vi "KM_FrequencyScan.vi"() -> ()   [LabVIEW 2015]
uses:
  MQM Data Transfer_KM.vi
  <vilib>/Utility/file.llb/Write To Spreadsheet File (string).vi
  <vilib>/Utility/file.llb/Write To Spreadsheet File (DBL).vi
  String Array Select.vi
  Numeric Array Select.vi
  plot refs -- filter related.ctl
  wavepacket.ctl
  filter method control.ctl
  peak -- parameters -- complex fit.ctl
  circle corners.ctl
  lorentzian.ctl
panel:
  out "cp lorentzian":T1={"Amplitude"=-1.0311345636926572, "omega(0)"=-1.0311345636926572, "Gamma"=-1.0311345636926572, "phase"=-1.0311345636926572, "Q"=-1.0311345636926572, "Norm  Ampl"=-1.0311345636926572, "z (inf)"=-1.0311345636926572+0.0i, "4corners"={"z (-pi/2)"=-1.0311345636926572+0.5736824521422934i, "z(inf)"=-0.5200164984937075+1.0975277942502903i, "z (pi/2)"=-1.0311345636926572+0.5736824521422934i, "z center"=-0.5136528600391839+0.580046090596817i, "z(0)"=-0.5200164984937075+1.0975277942502903i, "radius"=-1.0311345636926572}} {"z (inf)" format="%#9_9f"; "Q" format="%#9_9f"; "phase" format="%#9_9f"; "Gamma" format="%#9_9f"; "omega(0)" format="%#9_9f"}
  in  "subtract linear BG":bool
  in  "Tab Control":enum32{"Display Data", "Sweep Arming"}(tab)
  in  "Plot: fragment - filter":cluster{dbl[], dbl[]}[](graph)=[{array[953 elements], array[953 elements]}, {array[953 elements], array[953 elements]}, {array[953 elements], array[953 elements]}, {array[953 elements], array[953 elements]}]
  in  "scale gauge: Plot: complex plane - filter":dbl(slide)=0.00199 min=0.0 max=0.3 step=1e-05 scale=0.0001..0.3 scale format="%#_5g"
  in  "Plot: complex plane - filter":cluster{dbl[], dbl[]}[](graph)=[{array[953 elements], array[953 elements]}, {array[953 elements], array[953 elements]}, {[6.147901040838566e-05, 6.135373133876665e-05, 6.097838854916284e-05, 6.0354463346086974e-05, 5.948441807727129e-05, 5.837168641390595e-05, 5.702065979950748e-05, 5.54366701188976e-05, 5.362596865568959e-05, 5.1595701421327945e-05, 4.9353880953045816e-05, 4.690935469204115e-05, 4.427177006666834e-05, 4.145153641844591e-05, 3.8459783921141216e-05, 3.5308319655059415e-05, 3.200958100989166e-05, 2.8576586600020083e-05, 2.5022884885994518e-05, 2.1362500704948304e-05, 1.7609879920973602e-05, 1.3779832413895373e-05, 9.887473631441806e-06, 5.948164935477676e-06, 1.9774529777269755e-06, -2.0089916557587785e-06, -5.995436289244519e-06, -9.96614824699522e-06, -1.3905456942959363e-05, -1.779781572541292e-05, -2.1627863232491146e-05, -2.5380484016465848e-05, -2.904086819751206e-05, -3.259456991153764e-05, -3.6027564321409215e-05, -3.932630296657695e-05, -4.247776723265876e-05, -4.5469519729963454e-05, -4.8289753378185884e-05, -5.09273380035587e-05, -5.3371864264563346e-05, -5.561368473284548e-05, -5.764395196720713e-05, -5.945465343041514e-05, -6.103864311102503e-05, -6.238966972542349e-05, -6.350240138878883e-05, -6.437244665760451e-05, -6.499637186068038e-05, -6.537171465028419e-05, -6.54969937199032e-05, -6.537171465028419e-05, -6.499637186068038e-05, -6.437244665760451e-05, -6.350240138878883e-05, -6.238966972542349e-05, -6.103864311102501e-05, -5.945465343041513e-05, -5.764395196720712e-05, -5.5613684732845474e-05, -5.337186426456334e-05, -5.092733800355868e-05, -4.828975337818588e-05, -4.546951972996345e-05, -4.2477767232658746e-05, -3.9326302966576966e-05, -3.602756432140918e-05, -3.2594569911537626e-05, -2.904086819751202e-05, -2.5380484016465838e-05, -2.1627863232491146e-05, -1.7797815725412892e-05, -1.390545694295935e-05, -9.966148246995179e-06, -5.995436289244506e-06, -2.0089916557587802e-06, 1.9774529777270017e-06, 5.9481649354776745e-06, 9.887473631441845e-06, 1.3779832413895386e-05, 1.760987992097359e-05, 2.1362500704948328e-05, 2.5022884885994515e-05, 2.8576586600020124e-05, 3.200958100989167e-05, 3.5308319655059456e-05, 3.8459783921141236e-05, 4.145153641844591e-05, 4.427177006666836e-05, 4.690935469204116e-05, 4.9353880953045836e-05, 5.159570142132796e-05, 5.362596865568959e-05, 5.543667011889761e-05, 5.702065979950749e-05, 5.837168641390596e-05, 5.9484418077271304e-05, 6.0354463346086974e-05, 6.097838854916284e-05, 6.135373133876665e-05], [-1.1205323218261426e-05, -7.218878584775678e-06, -3.2481666270249814e-06, 6.911420689391552e-07, 4.583500851392718e-06, 8.413548358470941e-06, 1.2166169142445653e-05, 1.5826553323491864e-05, 1.938025503751744e-05, 2.2813249447389007e-05, 2.6111988092556765e-05, 2.9263452358638565e-05, 3.225520485594326e-05, 3.507543850416568e-05, 3.7713023129538496e-05, 4.015754939054316e-05, 4.239936985882529e-05, 4.442963709318694e-05, 4.6240338556394946e-05, 4.782432823700483e-05, 4.917535485140329e-05, 5.028808651476863e-05, 5.115813178358432e-05, 5.178205698666018e-05, 5.2157399776263995e-05, 5.2282678845883e-05, 5.2157399776263995e-05, 5.178205698666017e-05, 5.115813178358432e-05, 5.028808651476863e-05, 4.917535485140329e-05, 4.7824328237004825e-05, 4.624033855639494e-05, 4.4429637093186926e-05, 4.239936985882528e-05, 4.015754939054316e-05, 3.7713023129538496e-05, 3.5075438504165676e-05, 3.2255204855943246e-05, 2.926345235863855e-05, 2.611198809255677e-05, 2.2813249447389007e-05, 1.9380255037517432e-05, 1.5826553323491847e-05, 1.216616914244564e-05, 8.413548358470924e-06, 4.583500851392722e-06, 6.911420689391518e-07, -3.2481666270249915e-06, -7.218878584775692e-06, -1.1205323218261446e-05, -1.5191767851747172e-05, -1.9162479809497872e-05, -2.3101788505462016e-05, -2.6994147287915587e-05, -3.082419479499382e-05, -3.4576815578968526e-05, -3.8237199760014716e-05, -4.179090147404029e-05, -4.5223895883911866e-05, -4.852263452907963e-05, -5.167409879516143e-05, -5.466585129246611e-05, -5.7486084940688535e-05, -6.0123669566061355e-05, -6.2568195827066e-05, -6.481001629534815e-05, -6.684028352970978e-05, -6.865098499291781e-05, -7.023497467352768e-05, -7.158600128792615e-05, -7.26987329512915e-05, -7.356877822010717e-05, -7.419270342318303e-05, -7.456804621278685e-05, -7.469332528240585e-05, -7.456804621278685e-05, -7.419270342318303e-05, -7.356877822010717e-05, -7.269873295129148e-05, -7.158600128792615e-05, -7.023497467352767e-05, -6.86509849929178e-05, -6.684028352970978e-05, -6.481001629534813e-05, -6.256819582706598e-05, -6.0123669566061334e-05, -5.7486084940688535e-05, -5.4665851292466084e-05, -5.167409879516141e-05, -4.8522634529079576e-05, -4.522389588391184e-05, -4.179090147404029e-05, -3.823719976001468e-05, -3.45768155789685e-05, -3.0824194794993756e-05, -2.6994147287915553e-05, -2.310178850546201e-05, -1.9162479809497842e-05, -1.5191767851747167e-05]}, {[2.180843613001339e-05, -2.008991706602334e-06, -8.45318187396811e-06], [2.015688719802568e-05, -1.1205323149030123e-05, 1.4773194307782804e-05]}, {[3.113757403751932e-06, 2.0471841396985487e-06, 9.806108756451657e-07, -8.596238840821741e-08, -1.1525356524616005e-06, -2.2191089165149835e-06, -3.2856821805683666e-06, -4.35225544462175e-06, -5.418828708675133e-06, -6.485401972728517e-06, -7.551975236781899e-06, -8.618548500835281e-06, -9.685121764888665e-06, -1.0751695028942049e-05, -1.1818268292995431e-05, -1.2884841557048813e-05, -1.3951414821102197e-05, -1.5017988085155581e-05, -1.6084561349208965e-05, -1.7151134613262346e-05], [7.143908232533313e-06, 6.9167218796742506e-06, 6.689535526815188e-06, 6.462349173956126e-06, 6.235162821097064e-06, 6.0079764682380015e-06, 5.780790115378939e-06, 5.553603762519877e-06, 5.326417409660815e-06, 5.0992310568017525e-06, 4.87204470394269e-06, 4.644858351083628e-06, 4.417671998224566e-06, 4.1904856453655035e-06, 3.963299292506441e-06, 3.736112939647379e-06, 3.5089265867883167e-06, 3.2817402339292544e-06, 3.054553881070192e-06, 2.82736752821113e-06]}, {[-2.0089917066023344e-06, -9.360762157193256e-07, 1.3683927516368315e-07, 1.2097547660466921e-06, 2.2826702569297007e-06, 3.3555857478127092e-06, 4.428501238695719e-06, 5.501416729578727e-06, 6.574332220461736e-06, 7.647247711344744e-06, 8.720163202227753e-06, 9.793078693110761e-06, 1.0865994183993772e-05, 1.193890967487678e-05, 1.3011825165759789e-05, 1.4084740656642797e-05, 1.5157656147525806e-05, 1.6230571638408814e-05, 1.7303487129291823e-05, 1.837640262017483e-05], [-1.1205323149030123e-05, -1.1205323149030123e-05, -1.1205323149030123e-05, -1.1205323149030123e-05, -1.1205323149030123e-05, -1.1205323149030123e-05, -1.1205323149030123e-05, -1.1205323149030123e-05, -1.1205323149030123e-05, -1.1205323149030123e-05, -1.1205323149030123e-05, -1.1205323149030123e-05, -1.1205323149030123e-05, -1.1205323149030123e-05, -1.1205323149030123e-05, -1.1205323149030123e-05, -1.1205323149030123e-05, -1.1205323149030123e-05, -1.1205323149030123e-05, -1.1205323149030123e-05]}]
  out "Plot: dz/domega":cluster{"omega out":dbl[], dbl[]}(graph)
  out "Plot: win omega":T3(graph)
  out "Plot: phase":cluster{"omega out":dbl[], dbl[]}(graph)
  out "Plot: phase around center":cluster{dbl[], dbl[]}[](graph)
  out "Plot: fragment":cluster{dbl[], dbl[]}[](graph)
  out "Plot: complex plane":cluster{dbl[], dbl[]}[](graph)=[{array[953 elements], array[953 elements]}, {[3.0383024948080237e-05, 3.01580716927693e-05, 2.9486759574053305e-05, 2.8379675585066826e-05, 2.68542791016561e-05, 2.4934626537592202e-05, 2.2650991960555277e-05, 2.0039389652002364e-05, 1.714100614043495e-05, 1.4001550665240835e-05, 1.0670534314683625e-05, 7.200489206464318e-06, 3.646140024844015e-06, 6.354097968214359e-08, -3.4908082019381657e-06, -6.960853310157466e-06, -1.0291869660714675e-05, -1.3431325135908794e-05, -1.6329708647476206e-05, -1.8941310956029118e-05, -2.1224945533066037e-05, -2.314459809712994e-05, -2.4669994580540667e-05, -2.5777078569527143e-05, -2.6448390688243138e-05, -2.6673343943554075e-05, -2.6448390688243138e-05, -2.5777078569527143e-05, -2.466999458054066e-05, -2.3144598097129935e-05, -2.1224945533066034e-05, -1.8941310956029115e-05, -1.63297086474762e-05, -1.343132513590878e-05, -1.0291869660714658e-05, -6.960853310157466e-06, -3.49080820193816e-06, 6.354097968214909e-08, 3.646140024844027e-06, 7.200489206464335e-06, 1.0670534314683618e-05, 1.4001550665240833e-05, 1.7141006140434956e-05, 2.003938965200237e-05, 2.2650991960555284e-05, 2.4934626537592213e-05, 2.68542791016561e-05, 2.837967558506683e-05, 2.948675957405331e-05, 3.01580716927693e-05], [-2.50423120455284e-05, -2.1466782441215247e-05, -1.7947641074679964e-05, -1.454038690750597e-05, -1.1298754373304577e-05, -8.273865953597556e-06, -5.513425945744431e-06, -3.060968137675989e-06, -9.551692540527458e-07, 7.707609987872854e-07, 2.0896036697360487e-06, 2.9805598220342752e-06, 3.429578544928799e-06, 3.429578544928799e-06, 2.980559822034272e-06, 2.0896036697360487e-06, 7.70760998787282e-07, -9.551692540527492e-07, -3.060968137675989e-06, -5.513425945744438e-06, -8.273865953597552e-06, -1.129875437330458e-05, -1.4540386907505977e-05, -1.7947641074679964e-05, -2.146678244121525e-05, -2.504231204552841e-05, -2.8617841649841554e-05, -3.213698301637684e-05, -3.554423718355084e-05, -3.878586971775222e-05, -4.1810758137459246e-05, -4.4571198145312364e-05, -4.702365595338081e-05, -4.912945483700406e-05, -5.085538508984409e-05, -5.217422776079284e-05, -5.3065183913091077e-05, -5.35142026359856e-05, -5.35142026359856e-05, -5.306518391309107e-05, -5.217422776079285e-05, -5.085538508984409e-05, -4.912945483700405e-05, -4.7023655953380806e-05, -4.457119814531235e-05, -4.181075813745923e-05, -3.878586971775222e-05, -3.5544237183550826e-05, -3.213698301637683e-05, -2.8617841649841537e-05]}, {[-2.2995916620324662e-05, -2.051084090806589e-05, -1.8025765195807113e-05, -1.554068948354834e-05, -1.3055613771289565e-05, -1.057053805903079e-05, -8.085462346772018e-06, -5.600386634513241e-06, -3.1153109222544683e-06, -6.302352099956953e-07, 1.854840502263081e-06, 4.339916214521854e-06, 6.824991926780627e-06, 9.310067639039403e-06, 1.179514335129818e-05, 1.4280219063556949e-05, 1.6765294775815725e-05, 1.92503704880745e-05, 2.173544620033327e-05, 2.4220521912592048e-05], [-1.1031702558117846e-05, -1.2432763506858901e-05, -1.3833824455599956e-05, -1.5234885404341013e-05, -1.6635946353082066e-05, -1.8037007301823124e-05, -1.943806825056418e-05, -2.0839129199305234e-05, -2.224019014804629e-05, -2.3641251096787344e-05, -2.50423120455284e-05, -2.6443372994269454e-05, -2.7844433943010512e-05, -2.9245494891751567e-05, -3.064655584049262e-05, -3.2047616789233674e-05, -3.344867773797473e-05, -3.484973868671579e-05, -3.625079963545684e-05, -3.7651860584197894e-05]}, {[1.5865449989673634e-05, 1.4464389040932579e-05, 1.3063328092191524e-05, 1.1662267143450467e-05, 1.0261206194709412e-05, 8.860145245968358e-06, 7.459084297227301e-06, 6.058023348486246e-06, 4.656962399745191e-06, 3.255901451004136e-06, 1.854840502263081e-06, 4.5377955352202603e-07, -9.472813952190323e-07, -2.3483423439600873e-06, -3.7494032927011422e-06, -5.150464241442197e-06, -6.551525190183252e-06, -7.952586138924307e-06, -9.353647087665362e-06, -1.0754708036406417e-05], [-1.9155492294065947e-07, -2.6766306351994337e-06, -5.161706347458208e-06, -7.646782059716982e-06, -1.0131857771975756e-05, -1.2616933484234531e-05, -1.5102009196493304e-05, -1.758708490875208e-05, -2.0072160621010853e-05, -2.2557236333269626e-05, -2.5042312045528402e-05, -2.7527387757787175e-05, -3.0012463470045948e-05, -3.2497539182304725e-05, -3.49826148945635e-05, -3.746769060682227e-05, -3.995276631908105e-05, -4.243784203133982e-05, -4.492291774359859e-05, -4.740799345585737e-05]}, {[0.04673210164257447, 0.049919815487102684, 0.05307633107191166, 0.056199675677509844, 0.05928789731518806, 0.06233906594694866, 0.06535127469171664, 0.06832264101707818, 0.07125130791580202, 0.0741354450664087, 0.07697324997706184, 0.07976294911206679, 0.0825027990002728, 0.0851910873246857, 0.08782613399261033, 0.09040629218565366, 0.09292994938893286, 0.09539552839884442, 0.09780148830876523, 0.10014632547206899], [-0.12810601858774873, -0.1268978066952708, -0.12561028780431027, -0.1242442665722635, -0.12280059671793454, -0.12128018048798891, -0.11968396809307863, -0.11801295711399153, -0.11626819187819583, -0.11445076280716932, -0.11256180573492151, -0.11060250119813439, -0.10857407369836529, -0.10647779093677343, -0.10431496302184781, -0.10208694165063226, -0.09979511926395848, -0.09744092817621612, -0.09502583968020283, -0.09255136312761404]}, {[0.05358614321681127, 0.05724138842520362, 0.06086085962911791, 0.0644422947768705, 0.06798345558807486, 0.07148212895249367, 0.07493612831316095, 0.07834329503290884, 0.08170149974344551, 0.08500864367614118, 0.08826265997369011, 0.09146151498182913, 0.09460320952030535, 0.09768578013229881, 0.10070730031151905, 0.10366588170620873, 0.1065596752993022, 0.1093868725640008, 0.11214570659404333, 0.11483445320796498], [-0.1468949013139417, -0.145509485010567, -0.14403313001559898, -0.142466759002852, -0.14081135090322142, -0.13906794029288377, -0.13723761674671997, -0.13532152415736678, -0.13332086002032104, -0.13123687468554396, -0.12907087057603317, -0.1268242013738506, -0.12449827117411537, -0.12209453360749002, -0.11961449093170867, -0.11705969309271483, -0.11443173675599556, -0.11173226430871766, -0.10896296283328909, -0.10612556305298726]}, {array[953 elements], array[953 elements]}]
  in  "scale gauge: Plot: complex plane":dbl(slide)=0.08418000000000002 min=0.0 max=0.3 step=1e-05 scale=0.0001..1.0 scale format="%#_2g"
  in  "plot staff":enum16{"plot", "do not plot", "a"}(ring)=enum."do not plot"
  out "pm lorentzian":T1={"Amplitude"=0.000340055891053764, "omega(0)"=3392.560000065714, "Gamma"=11.91999763250351, "phase"=1.0574274315248449, "Q"=284.61079478865537, "Norm  Ampl"=nan, "z (inf)"=-2.2995916620324662e-05-1.1031702558117846e-05i, "4corners"={"z (-pi/2)"=1.5865449989673634e-05-1.9155492294065609e-07i, "z(inf)"=-2.2995916620324662e-05-1.1031702558117846e-05i, "z (pi/2)"=-1.2155768985147472e-05-4.9893069168116145e-05i, "z center"=1.8548405022630806e-06-2.50423120455284e-05i, "z(0)"=2.6705597624850824e-05-3.905292153293895e-05i, "radius"=2.8528184445817156e-05}} {"z (inf)" format="%#9_9f"; "Q" format="%#9_9f"; "phase" format="%#9_9f"; "Gamma" format="%#9_9f"; "omega(0)" format="%#9_9f"}
  in  "use fast fit?":bool=TRUE
  out "window width (kHz)":dbl=76.27809365793496
  out "window center (kHz)":dbl=3399.029286744401
  out "# of points in window":dbl=953.475933538175
  in  "parameters: complex fit":T4={"main VI path"=path "", "scale factor"=3.0, "# of grid points"=200, "parameters: wavepacket"={"R"=0.5, "wave number"=22.0, "delta k"=7.0, "radii vector"=[], "radial section"=[], "wave vector"=22.0, "wavepacket is"=TRUE}, "span"=0.27789, "interference ?"=enum."cp z center", "filter method"=enum."three"} {"span" min=0.0 max=0.5 step=1e-05 scale=0.0001..0.5 scale format="%#_5f"; "parameters: wavepacket"."delta k" format="%#_3f"; "parameters: wavepacket"."wave number" format="%#_3f"; "parameters: wavepacket"."R" format="%#_3f"}
  in  "Control":bool=TRUE
  in  "Stop":bool=TRUE
  out "XY Graph":cluster{dbl[], dbl[]}[](graph)
  in  "Display Elements":cluster{"X":bool, "Y":bool, "Name":u16}[](array[cluster]) {"Name" items=["Time (ms)", "Field (T)", "Temperature (K)", "", "HFLI_1.0 Freq (Hz)", "HFLI_1.0 R (V)", "HFLI_1.0 Theta (deg)", "HFLI_1.0 X (mV)", "HFLI_1.0 Y (mV)"]}
  in  "X-Axis":u16(ring) items=["Linear", "Reciprocal", "Log10"]
  in  "Filename":path=path "C:/Users/putkonen.CPFS/Dropbox.lvm"
  in  "Delay (ms)":dbl=2000.0
  out "Data Rate (ms)":u32
  in  "Finish":bool
  out "Measurement":bool
  in  "Y-Axis":u16(ring) items=["Linear", "Reciprocal", "Log10"]
  out "Saving":bool
  in  "Data Recording":bool=TRUE
  in  "DAQ time (ms)":u32=500
  out "Circles":cluster{dbl[], dbl[]}(graph)
  in  "X":u16(ring) items=["Linear", "Reciprocal", "Log10"]
  in  "Y":u16(ring) items=["Linear", "Reciprocal", "Log10"]
  out "Phase":cluster{dbl[], dbl[]}(graph)
  in  "Frequency":u16(ring) items=["Linear", "Reciprocal", "Log10"]
  in  "Theta":u16(ring) items=["Linear", "Reciprocal", "Log10"]
  out "# pts in freq sweep":i32
  out "Data Rate  (ms)":u32
  in  "DAQ time (ms)":u32=50
  in  "Fequency sweep datafile":path=path "C:/Users/putkonen.CPFS/Dropbox.lvm" caption="Filename"
  in  "Save current freq scan":bool
  in  "Start (Hz)":dbl=48.29
  in  "Stop (Hz)":dbl=48.57
  in  "# pts in scan":dbl=100.0
  in  "Bandwidth (Hz)":dbl=10.0
  out "good lorentzian":T1={"Amplitude"=-1.0311345636926572, "omega(0)"=-1.0311345636926572, "Gamma"=-1.0311345636926572, "phase"=-1.0311345636926572, "Q"=-1.0311345636926572, "Norm  Ampl"=-1.0311345636926572, "z (inf)"=-1.0311345636926572+0.0i, "4corners"={"z (-pi/2)"=-1.0311345636926572+0.5736824521422934i, "z(inf)"=-0.5200164984937075+1.0975277942502903i, "z (pi/2)"=-1.0311345636926572+0.5736824521422934i, "z center"=-0.5136528600391839+0.580046090596817i, "z(0)"=-0.5200164984937075+1.0975277942502903i, "radius"=-1.0311345636926572}} {"z (inf)" format="%#9_9f"; "Q" format="%#9_9f"; "phase" format="%#9_9f"; "Gamma" format="%#9_9f"; "omega(0)" format="%#9_9f"}
  in  "Use Sweep Control":bool
  in  "Sweep Parameter":u16(ring) items=["Temperature", "Field", "Position", "Measure when stable"]
  out "Global Stop":bool
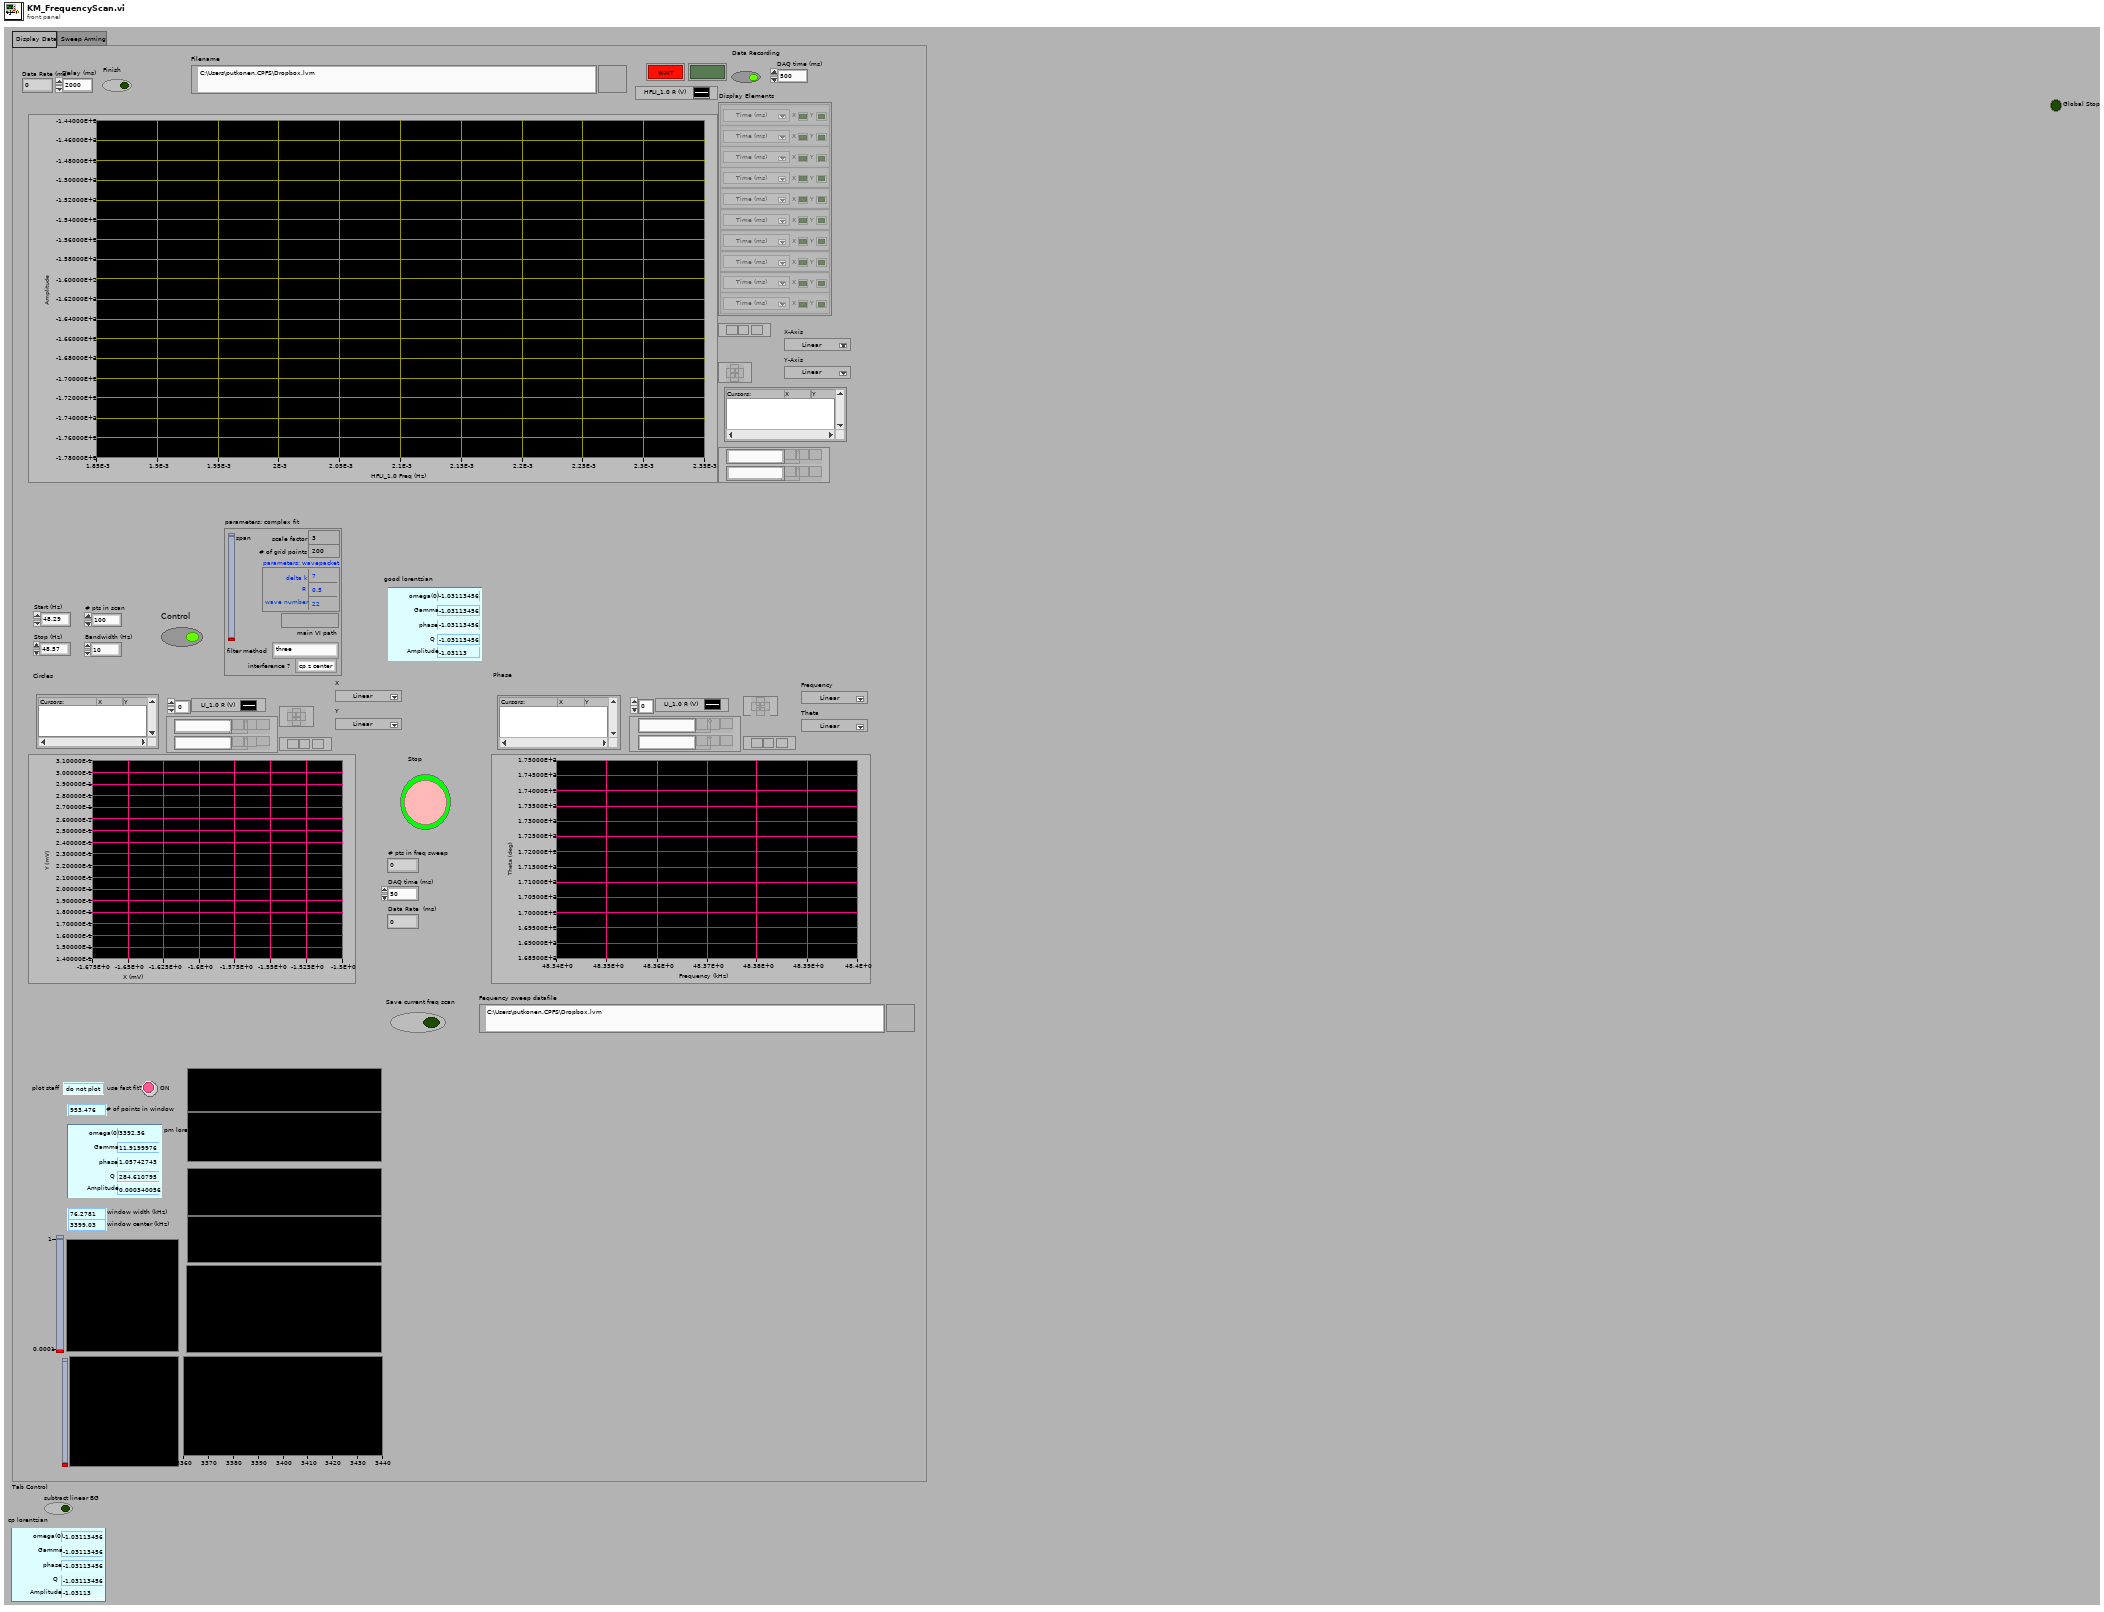
[diagram p1: front panel]
types:
  T1 = typedef "lorentzian.ctl" = cluster{"Amplitude":dbl, "omega(0)":dbl, "Gamma":dbl, "phase":dbl, "Q":dbl, "Norm  Ampl":dbl, "z (inf)":cdb, "4corners":T2}
  T2 = typedef "circle corners.ctl" = cluster{"z (-pi/2)":cdb, "z(inf)":cdb, "z (pi/2)":cdb, "z center":cdb, "z(0)":cdb, "radius":dbl}
  T3 = cluster{"omega out":dbl[], "win omega out":dbl[]}
  T4 = typedef "peak -- parameters -- complex fit.ctl" = cluster{"main VI path":path, "scale factor":dbl, "# of grid points":i32, "parameters: wavepacket":T5, "span":dbl, "interference ?":enum16{"cp z center", "pm zcenter", "fancy"}, "filter method":T6}
  T5 = typedef "wavepacket.ctl" = cluster{"R":dbl, "wave number":dbl, "delta k":dbl, "radii vector":dbl[], "radial section":cdb[], "wave vector":dbl, "wavepacket is":bool}
  T6 = typedef "filter method control.ctl" = enum16{"four", "five", "one", "two", "three", "zero", "minus one", "minus two"}
  T7 = typedef "plot refs -- filter related.ctl" = cluster{"Plot: complex plane - filter":refnum<vi>, "Plot: dz/domega":refnum<vi>, "Plot: fragment filter":refnum<vi>, "Plot: win omega":refnum<vi>, "Plot: phase":refnum<vi>, "Plot: phase around center":refnum<vi>, "Plot: complex plane":refnum<vi>, "Plot: fragment":refnum<vi>}
  T8 = typedef "ZI_Frontpanel.ctl" = cluster{"Lockin 1 Demod 0":cluster{"R(V)":dbl, "Theta (deg)":dbl, "Timestamp (ms)":u32}, "Lockin 2 Demod 0":cluster{"R(V)":dbl, "Theta (deg)":dbl, "Timestamp (ms)":u32}, "Lockin 3 Demod 0":cluster{"R(V)":dbl, "Theta (deg)":dbl, "Timestamp (ms)":u32}, "Lockin 4 Demod 0":cluster{"R(V)":dbl, "Theta (deg)":dbl, "Timestamp (ms)":u32}, "Lockin 1 Demod 1":cluster{"R(V)":dbl, "Theta (deg)":dbl, "Timestamp (ms)":u32}, "Lockin 2 Demod 1":cluster{"R(V)":dbl, "Theta (deg)":dbl, "Timestamp (ms)":u32}, "Lockin 3 Demod 1":cluster{"R(V)":dbl, "Theta (deg)":dbl, "Timestamp (ms)":u32}, "Lockin 4 Demod 1":cluster{"R(V)":dbl, "Theta (deg)":dbl, "Timestamp (ms)":u32}, "Lockin 1 Demod 2":cluster{"R(V)":dbl, "Theta (deg)":dbl, "Timestamp (ms)":u32}, "Lockin 1 Demod 3":cluster{"R(V)":dbl, "Theta (deg)":dbl, "Timestamp (ms)":u32}, "LI1 active":bool, "LI2 active":bool, "LI3 active":bool, "LI4 active":bool}
  T9 = typedef "PPMS_Status.ctl" = cluster{"Field":cluster{"Field (T)":dbl, "Field stable":bool, "Timestamp (ms)":u32}, "Temperature":cluster{"Temperature (K)":dbl, "Temperature stable":bool, "Timestamp (ms)":u32}}
  T10 = typedef "Rotator_Status.ctl" = cluster{"Angle (deg)":dbl, "Stopped":bool, "Timestamp (ms)":u32}
  T11 = cluster{"Request new file":bool, "Sweep variable":u16, "Pause DAQ":bool}
  T12 = typedef "HF_FrontPanel.ctl" = cluster{"Lockin 1 Demod 0":cluster{"R(V)":dbl, "Theta (deg)":dbl, "Frequency (Hz)":dbl, "X (mV)":dbl, "Y (mV)":dbl}, "LI1 active":bool, "Timestamp (ms)":u32}
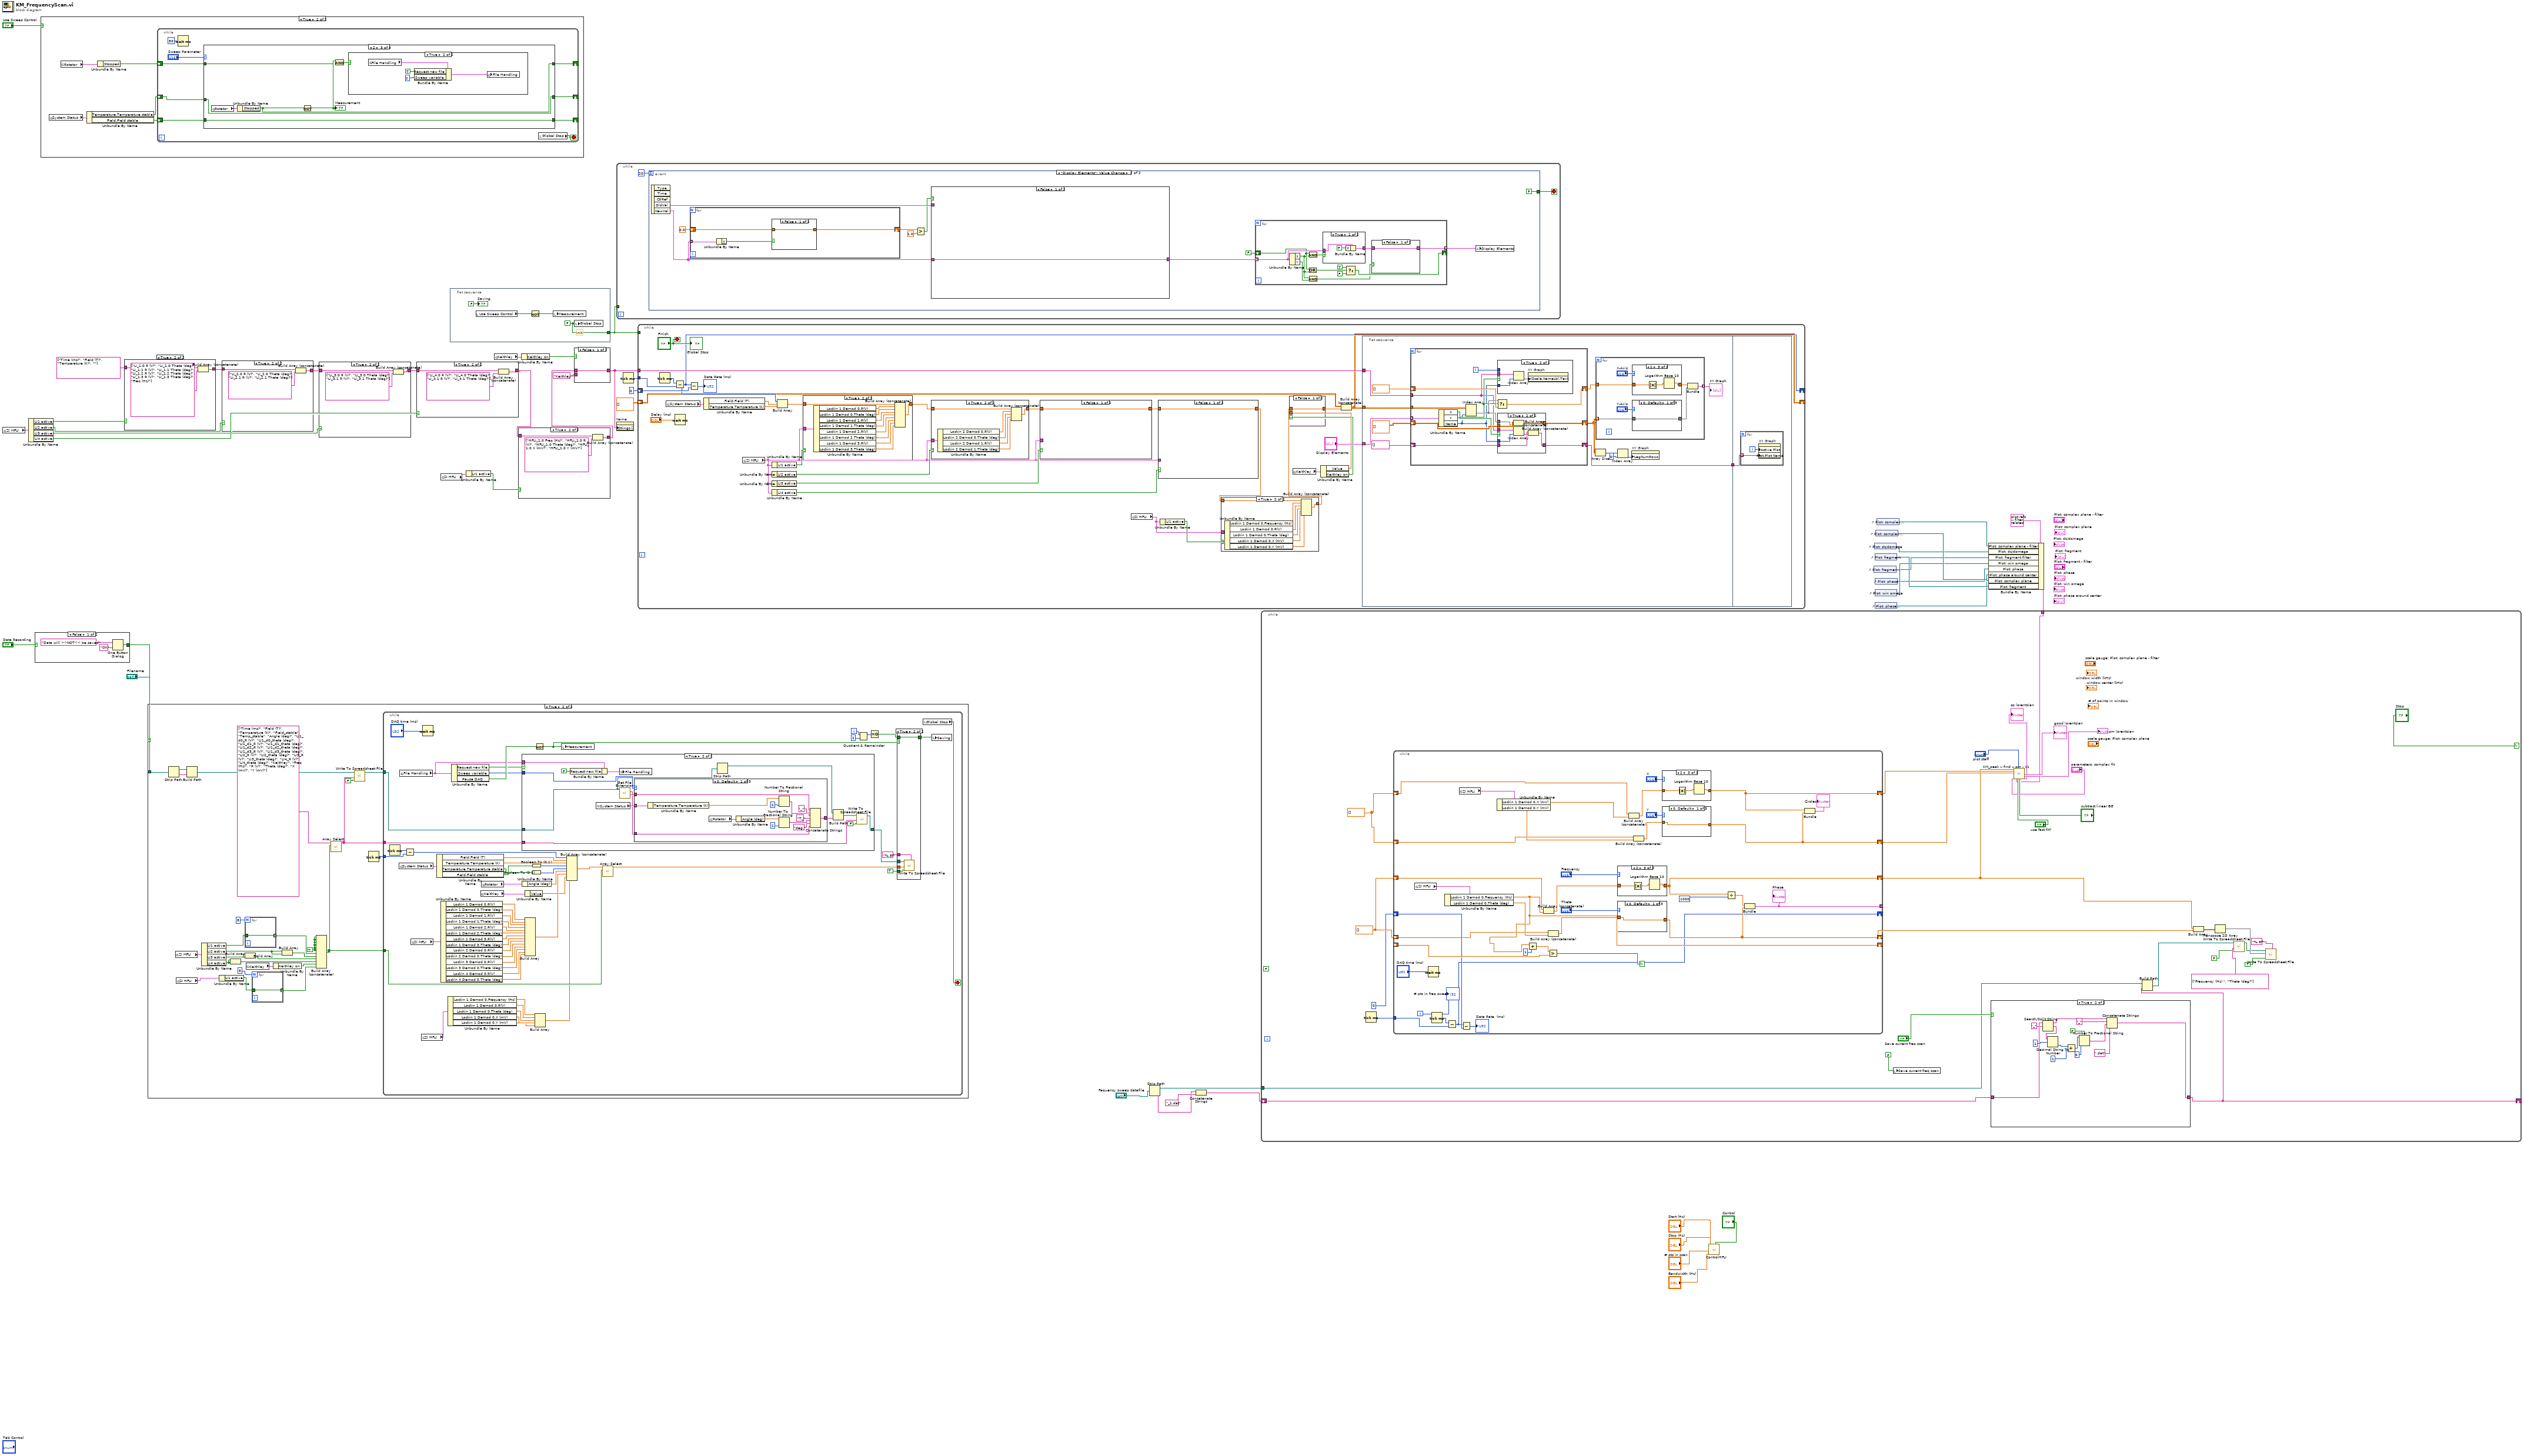
[diagram p0: block diagram]
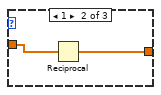
[diagram p3: hidden frame]
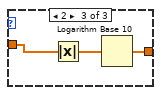
[diagram p4: hidden frame]
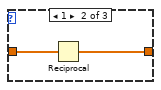
[diagram p6: hidden frame]
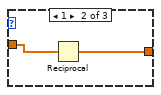
[diagram p7: hidden frame]
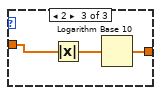
[diagram p8: hidden frame]
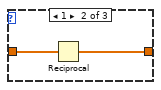
[diagram p10: hidden frame]
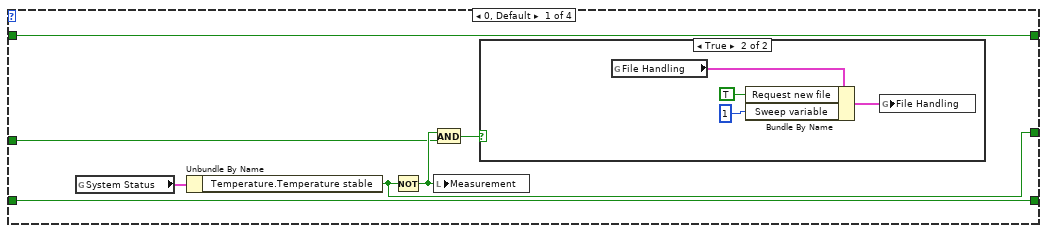
[diagram p13: hidden frame]
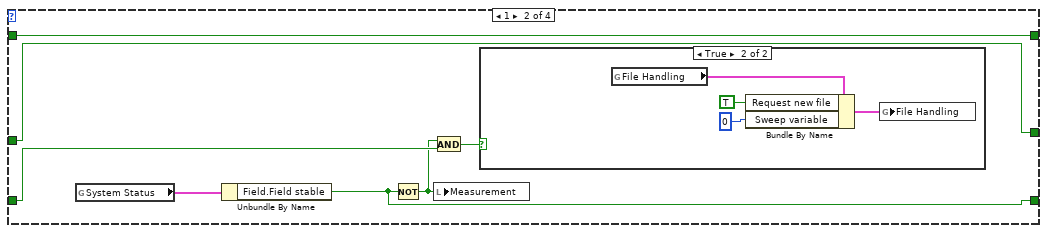
[diagram p15: hidden frame]
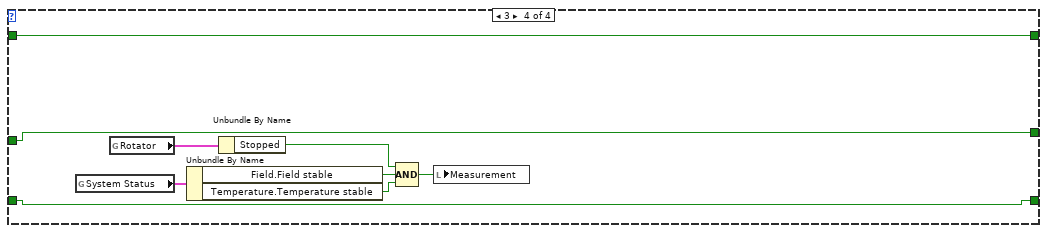
[diagram p18: hidden frame]
diagram:
  n1 = global read "MQM Data Transfer_KM.vi" "ZI MFLI"() -> (w43:T8)
  n2 = Unbundle By Name(w43) -> ("LI1 active"=w42:bool, "LI2 active"=w40:bool, "LI3 active"=w34:bool, "LI4 active"=w33:bool)
  n3 = case shown="False" "Data Recording" {
    selector: "Data Recording" -> [_ w49]
    tunnel: [w46 w49] -> w27
    frame False {
      n4 = One Button Dialog(message="Data will >>NOT<< be saved", button name ("OK")="OK") -> (true=w46:bool)
    }
    frame True {
    }
  }
  n5 = case shown="True" "Use Sweep Control" {
    frame False {
    }
    frame True {
      n6 = global read "MQM Data Transfer_KM.vi" "System Status"() -> (w52:T9)
      n7 = global read "MQM Data Transfer_KM.vi" "Rotator"() -> (w54:T10)
      n8 = Unbundle By Name(w52) -> ("Temperature.Temperature stable"=w51:bool, "Field.Field stable"=w50:bool)
      n9 = Unbundle By Name(w54) -> ("Stopped"=w53:bool)
      n10 = while {
        shift-right: [w61] -> _
        shift-left: w53 -> [w60]
        shift-right: [w58] -> _
        shift-left: w51 -> [w59]
        shift-right: [w57] -> _
        shift-left: w50 -> [w56]
        stop <- w55 stop-if-true
        n11 = Wait (ms)(milliseconds to wait=u32 50) -> ()  [unwired: 1 out]
        n12 = case shown="2" "Sweep Parameter" {
          tunnel: [w69 w79 w91 w99] -> w61
          tunnel: w60 -> [w69 w79 w89 w99]
          tunnel: w59 -> [w66 w80 w87 w98]
          tunnel: [w68 w80 w87 w98] -> w58
          tunnel: [w64 w76 w86 w97] -> w57
          tunnel: w56 -> [w64 w77 w86 w97]
          frame 0, Default {
            n13 = global read "MQM Data Transfer_KM.vi" "System Status"() -> (w70:T9)
            n14 = Unbundle By Name(w70) -> ("Temperature.Temperature stable"=w68:bool)
            n15 = Not(x=w68) -> (.not. x?=w67:bool)
            n16 = And(x=w67, y=w66) -> (x .and. y?=w65:bool)
            n17 = local write "Measurement"(w67) -> ()
            n18 = case shown="True" w65 {
              frame False {
              }
              frame True {
                n19 = global read "MQM Data Transfer_KM.vi" "File Handling"() -> (w74:T11)
                n20 = Bundle By Name(cluster=w74, "Request new file"=TRUE, "Sweep variable"=u16 1) -> (w73:T11)
                n21 = global write "MQM Data Transfer_KM.vi" "File Handling"(w73) -> ()
              }
            }
          }
          frame 1 {
            n22 = global read "MQM Data Transfer_KM.vi" "System Status"() -> (w81:T9)
            n23 = Unbundle By Name(w81) -> ("Field.Field stable"=w76:bool)
            n24 = Not(x=w76) -> (.not. x?=w75:bool)
            n25 = And(x=w75, y=w77) -> (x .and. y?=w78:bool)
            n26 = local write "Measurement"(w75) -> ()
            n27 = case shown="True" w78 {
              frame False {
              }
              frame True {
                n28 = global read "MQM Data Transfer_KM.vi" "File Handling"() -> (w85:T11)
                n29 = Bundle By Name(cluster=w85, "Request new file"=TRUE, "Sweep variable"=u16 0) -> (w84:T11)
                n30 = global write "MQM Data Transfer_KM.vi" "File Handling"(w84) -> ()
              }
            }
          }
          frame 2 {
            n31 = global read "MQM Data Transfer_KM.vi" "Rotator"() -> (w92:T10)
            n32 = Unbundle By Name(w92) -> ("Stopped"=w91:bool)
            n33 = Not(x=w91) -> (.not. x?=w90:bool)
            "Measurement" <- w90
            n34 = And(x=w90, y=w89) -> (x .and. y?=w88:bool)
            n35 = case shown="True" w88 {
              frame False {
              }
              frame True {
                n36 = global read "MQM Data Transfer_KM.vi" "File Handling"() -> (w96:T11)
                n37 = Bundle By Name(cluster=w96, "Request new file"=TRUE, "Sweep variable"=u16 2) -> (w95:T11)
                n38 = global write "MQM Data Transfer_KM.vi" "File Handling"(w95) -> ()
              }
            }
          }
          frame 3 {
            n39 = global read "MQM Data Transfer_KM.vi" "System Status"() -> (w103:T9)
            n40 = global read "MQM Data Transfer_KM.vi" "Rotator"() -> (w105:T10)
            n41 = Unbundle By Name(w103) -> ("Field.Field stable"=w102:bool, "Temperature.Temperature stable"=w101:bool)
            n42 = Unbundle By Name(w105) -> ("Stopped"=w104:bool)
            n43 = Compound Arithmetic op=AND(w104, w102, w101) -> (w100:bool)
            n44 = local write "Measurement"(w100) -> ()
          }
        }
        n45 = local read "Global Stop"() -> (w55:bool)
      }
    }
  }
  n46 = case shown="True" w42 {
    tunnel: string[] ["Time (ms)", "Field (T)", "Temperature (K)", ""] -> [w106 w109]
    tunnel: [w106 w107] -> w39
    frame False {
    }
    frame True {
      n47 = Build Array (concatenate)(w109, string[] ["LI_1.0 R (V)", "LI_1.0 Theta (deg)", "LI_1.1 R (V)", "LI_1.1 Theta (deg)", "LI_1.2 R (V)", "LI_1.2 Theta (deg)", "LI_1.3 R (V)", "LI_1.3 Theta (deg)", "Freq (Hz)"]) -> (w107:string[])
    }
  }
  n48 = case shown="True" w27 {
    tunnel: "Filename" -> [_ w136]
    frame False {
    }
    frame True {
      w128 = TRUE
      n49 = Strip Path(path=w136) -> (stripped path=w132:path, name=w130:string)
      n50 = global read "MQM Data Transfer_KM.vi" "ZI MFLI"() -> (w127:T8)
      n51 = global read "MQM Data Transfer_KM.vi" "ZI HFLI"() -> (w113:T12)
      n52 = Build Path(base path=w132, name or relative path=w130) -> (appended path=w133:path)
      n53 = Unbundle By Name(w127) -> ("LI1 active"=w126:bool, "LI2 active"=w123:bool, "LI3 active"=w122:bool, "LI4 active"=w121:bool)
      n54 = Unbundle By Name(w113) -> ("LI1 active"=w112:bool)
      n55 = Build Array(w121, w121) -> (w118:bool[])
      n56 = for {
        N: 8 -> [_]
        tunnel: w126 -> [w138]
        tunnel: [w138] -> w124 mode=indexing
      }
      n57 = Build Array(w122, w122) -> (w119:bool[])
      n58 = global read "MQM Data Transfer_KM.vi" "Keithley"() -> (w117:cluster{"Value":dbl, "Keithley on":bool})
      n59 = for {
        N: 5 -> [_]
        tunnel: w112 -> [w137]
        tunnel: [w137] -> w110 mode=indexing
      }
      n60 = Unbundle By Name(w117) -> ("Keithley on"=w116:bool)
      n61 = Build Array(w123, w123) -> (w120:bool[])
      n62 = Build Array (concatenate)(w128, w128, w128, w128, w128, w128, w124, w120, w119, w118, w116, w110) -> (w115:bool[])
      n63 = call-poly "Array Select.vi"("Selector array"=w115, "Full array"=string[] ["Time (ms)", "Field (T)", "Temperature (K)", "Field_stable", "Temp_stable", "Angle (deg)", "LI1_d0_R (V)", "LI1_d0_theta (deg)", "LI1_d1_R (V)", "LI1_d1_theta (deg)", "LI1_d2_R (V)", "LI1_d2_theta (deg)", "LI1_d3_R (V)", "LI1_d3_theta (deg)", "LI2_R (V)", "LI2_theta (deg)", "LI3_R (V)", "LI3_theta (deg)", "LI4_R (V)", "LI4_theta (deg)", "Keithley", "Freq (Hz)", "R (V)", "Theta (deg)", "X (mV)", "Y (mV)"]) -> ("Array"=w114:string[])  [unwired: 9 in]
      n64 = call-poly <vilib>:"Write To Spreadsheet File.vi"("append to file? (new file:F)"=FALSE, "1D data"=w114, "file path (dialog if empty)"=w133) -> ("new file path (Not A Path if cancelled)"=w131:path)  [unwired: 5 in]
      n65 = Tick Count (ms)() -> (millisecond timer value=w135:u32)
      n66 = while {
        tunnel: w135 -> [w195]
        tunnel: w131 -> [w153]
        tunnel: w115 -> [w162]
        tunnel: w114 -> [w150]
        i -> [w161]
        stop <- w187 stop-if-true
        n67 = Tick Count (ms)() -> (millisecond timer value=w193:u32)
        n68 = global read "MQM Data Transfer_KM.vi" "System Status"() -> (w194:T9)
        n69 = global read "MQM Data Transfer_KM.vi" "File Handling"() -> (w149:T11)
        n70 = Subtract(x=w193, y=w195) -> (x-y=w192:u32)
        n71 = global read "MQM Data Transfer_KM.vi" "ZI MFLI"() -> (w183:T8)
        n72 = global read "MQM Data Transfer_KM.vi" "ZI HFLI"() -> (w146:T12)
        n73 = Wait (ms)(milliseconds to wait="DAQ time (ms)") -> ()  [unwired: 1 out]
        n74 = Unbundle By Name(w194) -> ("Field.Field (T)"=w191:dbl, "Temperature.Temperature (K)"=w190:dbl, "Temperature.Temperature stable"=w171:bool, "Field.Field stable"=w173:bool)
        n75 = Unbundle By Name(w183) -> ("Lockin 1 Demod 0.R(V)"=w182:dbl, "Lockin 1 Demod 0.Theta (deg)"=w181:dbl, "Lockin 1 Demod 1.R(V)"=w180:dbl, "Lockin 1 Demod 1.Theta (deg)"=w179:dbl, "Lockin 1 Demod 2.R(V)"=w178:dbl, "Lockin 1 Demod 2.Theta (deg)"=w177:dbl, "Lockin 1 Demod 3.R(V)"=w176:dbl, "Lockin 1 Demod 3.Theta (deg)"=w175:dbl, "Lockin 2 Demod 0.R(V)"=w174:dbl, "Lockin 2 Demod 0.Theta (deg)"=w167:dbl, "Lockin 3 Demod 0.R(V)"=w166:dbl, "Lockin 3 Demod 0.Theta (deg)"=w165:dbl, "Lockin 4 Demod 0.R(V)"=w164:dbl, "Lockin 4 Demod 0.Theta (deg)"=w163:dbl)
        n76 = Unbundle By Name(w146) -> ("Lockin 1 Demod 0.Frequency (Hz)"=w145:dbl, "Lockin 1 Demod 0.R(V)"=w144:dbl, "Lockin 1 Demod 0.Theta (deg)"=w143:dbl, "Lockin 1 Demod 0.X (mV)"=w142:dbl, "Lockin 1 Demod 0.Y (mV)"=w141:dbl)
        n77 = Unbundle By Name(w149) -> ("Request new file"=w154:bool, "Sweep variable"=w151:u16, "Pause DAQ"=w158:bool)
        n78 = global read "MQM Data Transfer_KM.vi" "Keithley"() -> (w184:cluster{"Value":dbl, "Keithley on":bool})
        n79 = global read "MQM Data Transfer_KM.vi" "Rotator"() -> (w185:T10)
        n80 = case shown="True" w154 {
          tunnel: w153 -> [w196 w207]
          tunnel: [w196 w200] -> w152
          tunnel: w151 -> [_ w209]
          tunnel: w150 -> [_ w202]
          tunnel: w149 -> [_ w199]
          frame False {
          }
          frame True {
            n81 = Bundle By Name(cluster=w199, "Request new file"=FALSE) -> (w197:T11)
            n82 = global read "MQM Data Transfer_KM.vi" "System Status"() -> (w208:T9)
            n83 = global write "MQM Data Transfer_KM.vi" "File Handling"(w197) -> ()
            n84 = call <vilib>:"Get File Extension.vi"("file"=w207) -> ("filename without extension"=w206:string, "lowercase file extension"=w205:string)  [unwired: 6 in, 3 out]
            n85 = case shown="0, Default" w209 {
              tunnel: w208 -> [w224 w233 w244]
              tunnel: w206 -> [w221 w234 w246]
              tunnel: w205 -> [w211 w225 w239]
              tunnel: [w217 w231 w245] -> w204
              frame 0, Default {
                n86 = Unbundle By Name(w224) -> ("Temperature.Temperature (K)"=w223:dbl)
                n87 = global read "MQM Data Transfer_KM.vi" "Rotator"() -> (w216:T10)
                n88 = Unbundle By Name(w216) -> ("Angle (deg)"=w214:dbl)
                n89 = Number To Fractional String(number=w223, precision (6)=i16 2) -> (F-format string=w219:string)  [unwired: 2 in]
                n90 = Number To Fractional String(number=w214, precision (6)=i16 1) -> (F-format string=w213:string)  [unwired: 2 in]
                n91 = Concatenate Strings(w221, "_", w219, "T_", w213, "deg." ("string"), w211) -> (w217:string)
              }
              frame 1 {
                n92 = Unbundle By Name(w233) -> ("Field.Field (T)"=w232:dbl)
                n93 = global read "MQM Data Transfer_KM.vi" "Rotator"() -> (w230:T10)
                n94 = Unbundle By Name(w230) -> ("Angle (deg)"=w228:dbl)
                n95 = Number To Fractional String(number=w232, precision (6)=i16 2) -> (F-format string=w236:string)  [unwired: 2 in]
                n96 = Number To Fractional String(number=w228, precision (6)=i16 1) -> (F-format string=w227:string)  [unwired: 2 in]
                n97 = Concatenate Strings(w234, "_", w236, "T_", w227, "deg." ("string"), w225) -> (w231:string)
              }
              frame 2 {
                n98 = Unbundle By Name(w244) -> ("Field.Field (T)"=w251:dbl, "Temperature.Temperature (K)"=w242:dbl)
                n99 = Number To Fractional String(number=w251, precision (6)=i16 2) -> (F-format string=w248:string)  [unwired: 2 in]
                n100 = Number To Fractional String(number=w242, precision (6)=i16 2) -> (F-format string=w241:string)  [unwired: 2 in]
                n101 = Concatenate Strings(w246, "_", w248, "T_", w241, "K." ("string"), w239) -> (w245:string)
              }
            }
            n102 = Strip Path(path=w207) -> (stripped path=w210:path)  [unwired: 1 out]
            n103 = Build Path(base path=w210, name or relative path=w204) -> (appended path=w201:path)
            n104 = call-poly <vilib>:"Write To Spreadsheet File.vi"("append to file? (new file:F)"=FALSE, "1D data"=w202, "file path (dialog if empty)"=w201) -> ("new file path (Not A Path if cancelled)"=w200:path)  [unwired: 5 in]
          }
        }
        n105 = Unbundle By Name(w185) -> ("Angle (deg)"=w169:dbl)
        n106 = Build Array(w182, w181, w180, w179, w178, w177, w176, w175, w174, w167, w166, w165, w164, w163) -> (w168:dbl[])
        n107 = Unbundle By Name(w184) -> ("Value"=w147:dbl)
        n108 = Boolean To (0,1)(Boolean=w173) -> (0, 1=w172:i16)
        n109 = Boolean To (0,1)(Boolean=w171) -> (0, 1=w170:i16)
        n110 = Not(x=w158) -> (.not. x?=w157:bool)
        n111 = Build Array(w145, w144, w143, w142, w141) -> (w140:dbl[])
        n112 = local write "Measurement"(w157) -> ()
        n113 = Build Array (concatenate)(w192, w191, w190, w172, w170, w169, w168, w147, w140) -> (w148:dbl[])
        n114 = call-poly "Array Select.vi"("Selector array"=w162, "Full array"=w148) -> ("Array"=w139:dbl[])  [unwired: 9 in]
        n115 = Quotient & Remainder(x=w161, y=2) -> (x-y*floor(x/y)=w159:i32)  [unwired: 1 out]
        n116 = Equal To 0?(x=w159) -> (x = 0?=w156:bool)
        n117 = case shown="True" w157 {
          tunnel: TRUE ("append to file? (new file:F)") -> [_ w257]
          tunnel: "%.8f" ("format (%.3f)") -> [_ w256]
          tunnel: w139 -> [_ w255]
          tunnel: w156 -> [_ w254]
          tunnel: [FALSE w254] -> w155
          tunnel: w152 -> [_ w253]
          frame False {
          }
          frame True {
            n118 = call-poly <vilib>:"Write To Spreadsheet File.vi"("format (%.3f)"=w256, "append to file? (new file:F)"=w257, "1D data"=w255, "file path (dialog if empty)"=w253) -> ()  [unwired: 4 in, 1 out]
          }
        }
        n119 = local read "Global Stop"() -> (w187:bool)
        n120 = local write "Saving"(w155) -> ()
      }
    }
  }
  n121 = case shown="True" w40 {
    tunnel: w39 -> [w258 w261]
    tunnel: [w258 w259] -> w38
    frame False {
    }
    frame True {
      n122 = Build Array (concatenate)(w261, string[] ["LI_2.0 R (V)", "LI_2.0 Theta (deg)", "LI_2.1 R (V)", "LI_2.1 Theta (deg)"]) -> (w259:string[])
    }
  }
  n123 = case shown="True" w34 {
    tunnel: w38 -> [w262 w265]
    tunnel: [w262 w263] -> w37
    frame False {
    }
    frame True {
      n124 = Build Array (concatenate)(w265, string[] ["LI_3.0 R (V)", "LI_3.0 Theta (deg)", "LI_3.1 R (V)", "LI_3.1 Theta (deg)"]) -> (w263:string[])
    }
  }
  n125 = case shown="True" w33 {
    tunnel: w37 -> [w266 w269]
    tunnel: [w266 w268] -> w22
    frame False {
    }
    frame True {
      n126 = Build Array (concatenate)(w269, string[] ["LI_4.0 R (V)", "LI_4.0 Theta (deg)", "LI_4.1 R (V)", "LI_4.1 Theta (deg)"]) -> (w268:string[])
    }
  }
  n127 = global read "MQM Data Transfer_KM.vi" "ZI HFLI"() -> (w24:T12)
  n128 = flat-sequence {
    tunnel: [w273] -> w35
    frame #0 {
      w273 = FALSE ("Global Stop")
      # "Init"
      n129 = local read "Use Sweep Control"() -> (w271:bool)
      n130 = Not(x=w271) -> (.not. x?=w270:bool)
      n131 = local write "Measurement"(w270) -> ()
      n132 = local write "Global Stop"(w273) -> ()
      "Saving" <- FALSE ("Saving")
    }
  }
  n133 = Unbundle By Name(w24) -> ("LI1 active"=w23:bool)
  n134 = global read "MQM Data Transfer_KM.vi" "Keithley"() -> (w30:cluster{"Value":dbl, "Keithley on":bool})
  n135 = case shown="True" w23 {
    tunnel: w22 -> [w274 w277]
    tunnel: [w274 w275] -> w21
    frame False {
    }
    frame True {
      n136 = Build Array (concatenate)(w277, string[] ["HFLI_1.0 Freq (Hz)", "HFLI_1.0 R (V)", "HFLI_1.0 Theta (deg)", "HFLI_1.0 X (mV)", "HFLI_1.0 Y (mV)"]) -> (w275:string[])
    }
  }
  n137 = Unbundle By Name(w30) -> ("Keithley on"=w29:bool)
  n138 = case shown="False" w29 {
    tunnel: w21 -> [w278 w281]
    tunnel: "Keithley" -> [_ w280]
    tunnel: [w278 w279] -> w31
    frame False {
    }
    frame True {
      n139 = Build Array (concatenate)(w281, w280) -> (w279:string[])
    }
  }
  n140 = while {
    tunnel: w35 -> [_]
    stop <- w282 stop-if-true
    n141 = event shown="[1] \"Display Elements\": Value Change" {
      selector: _ -> [_ _]
      dyn-events: _ -> [_ _]
      timeout: 20 -> [_ _]
      tunnel: [w284 FALSE] -> w282
      event Timeout {
        n142 = event-data() -> ()  [unwired: 1 in, 2 out]
        n143 = local read "Global Stop"() -> (w285:bool)
        n144 = case shown="False" w285 {
          tunnel: [FALSE TRUE] -> w284
          frame False {
          }
          frame True {
          }
        }
      }
      event "Display Elements": Value Change {
        n145 = event-data() -> ("OldVal"=w295:cluster{"X":bool, "Y":bool, "Name":u16}[], "NewVal"=w293:cluster{"X":bool, "Y":bool, "Name":u16}[])  [unwired: 1 in, 3 out]
        n146 = for {
          tunnel: w293 -> [w318] mode=indexing
          shift-right: [w316] -> w291
          shift-left: 0.0 -> [w315]
          n147 = Unbundle By Name(w318) -> ("X"=w317:bool)
          n148 = case shown="False" w317 {
            tunnel: [w319 w321] -> w316
            tunnel: w315 -> [w319 w320]
            frame False {
            }
            frame True {
              n149 = Increment(x=w320) -> (x+1=w321:dbl)
            }
          }
        }
        n150 = Greater?(x=w291, y=1.0) -> (0:w289:bool)
        n151 = case shown="False" w289 {
          tunnel: w295 -> [_ w301]
          tunnel: [w298 w300] -> w294
          tunnel: w293 -> [w298 w299]
          frame False {
          }
          frame True {
            n152 = for {
              tunnel: w299 -> [w304] mode=indexing
              tunnel: w301 -> [w308] mode=indexing
              tunnel: [w303] -> w300 mode=indexing
              n153 = Unbundle By Name(w308) -> ("X"=w307:bool)
              n154 = Unbundle By Name(w304) -> ("X"=w306:bool)
              n155 = Not(x=w307) -> (.not. x?=w305:bool)
              n156 = And(x=w305, y=w306) -> (x .and. y?=w302:bool)
              n157 = case shown="True" w302 {
                tunnel: [w309 w313] -> w303
                tunnel: w304 -> [w311 w312]
                frame False {
                  n158 = Bundle By Name(cluster=w311, "X"=FALSE) -> (w309:cluster{"X":bool, "Y":bool, "Name":u16})
                }
                frame True {
                  n159 = Bundle By Name(cluster=w312, "X"=TRUE) -> (w313:cluster{"X":bool, "Y":bool, "Name":u16})
                }
              }
            }
          }
        }
        n160 = for {
          tunnel: w294 -> [w332] mode=indexing
          shift-right: [w328] -> _
          shift-left: FALSE ("X") -> [w331]
          tunnel: [w322] -> w296 mode=indexing
          n161 = Unbundle By Name(w332) -> ("X"=w326:bool, "Y"=w325:bool)
          n162 = Or(x=w331, y=w326) -> (x .or. y?=w330:bool)
          n163 = And(x=w331, y=w326) -> (x .and. y?=w333:bool)
          n164 = And(x=w326, y=w325) -> (x .and. y?=w324:bool)
          n165 = case shown="True" w333 {
            tunnel: w332 -> [w338 w341]
            tunnel: [w338 w339] -> w323
            frame False {
            }
            frame True {
              n166 = Bundle By Name(cluster=w341, "X"=FALSE) -> (w339:cluster{"X":bool, "Y":bool, "Name":u16})
            }
          }
          n167 = Select(t=TRUE, s=w330, f=FALSE) -> (s? t:f=w328:bool)
          n168 = case shown="False" w324 {
            tunnel: w323 -> [w334 w337]
            tunnel: [w334 w336] -> w322
            frame False {
            }
            frame True {
              n169 = Bundle By Name(cluster=w337, "Y"=FALSE) -> (w336:cluster{"X":bool, "Y":bool, "Name":u16})
            }
          }
        }
        n170 = local write "Display Elements"(w296) -> ()
      }
    }
  }
  n171 = property on="Name" class="Ring (strict)"("Strings []"=w31) -> ()  [unwired: 2 in, 2 out]
  n172 = Tick Count (ms)() -> (millisecond timer value=w45:u32)
  n173 = while {
    tunnel: w45 -> [w372]
    shift-right: [w363] -> _
    shift-left: 0 -> [w371]
    tunnel: w31 -> [w365]
    shift-right: [w350] -> _
    shift-left: dbl[][] [] -> [w351]
    tunnel: w35 -> [_]
    stop <- "Finish" stop-if-true
    n174 = Tick Count (ms)() -> (millisecond timer value=w373:u32)
    n175 = global read "MQM Data Transfer_KM.vi" "System Status"() -> (w354:T9)
    n176 = Subtract(x=w373, y=w372) -> (x-y=w363:u32)
    n177 = Wait (ms)(milliseconds to wait="Delay (ms)") -> ()  [unwired: 1 out]
    n178 = Subtract(x=w363, y=w371) -> (x-y=→"Data Rate (ms)":u32)
    n179 = Unbundle By Name(w354) -> ("Field.Field (T)"=w353:dbl, "Temperature.Temperature (K)"=w352:dbl)
    n180 = global read "MQM Data Transfer_KM.vi" "ZI MFLI"() -> (w356:T8)
    n181 = Unbundle By Name(w356) -> ("LI1 active"=w364:bool)
    n182 = Unbundle By Name(w356) -> ("LI2 active"=w361:bool)
    n183 = Unbundle By Name(w356) -> ("LI3 active"=w359:bool)
    n184 = Unbundle By Name(w356) -> ("LI4 active"=w357:bool)
    n185 = Build Array(w363, w353, w352) -> (w362:dbl[])
    n186 = case shown="True" w364 {
      tunnel: w356 -> [_ w422]
      tunnel: w362 -> [w411 w421]
      tunnel: [w411 w412] -> w360
      frame False {
      }
      frame True {
        n187 = Unbundle By Name(w422) -> ("Lockin 1 Demod 0.R(V)"=w420:dbl, "Lockin 1 Demod 0.Theta (deg)"=w419:dbl, "Lockin 1 Demod 1.R(V)"=w418:dbl, "Lockin 1 Demod 1.Theta (deg)"=w417:dbl, "Lockin 1 Demod 2.R(V)"=w416:dbl, "Lockin 1 Demod 2.Theta (deg)"=w415:dbl, "Lockin 1 Demod 3.R(V)"=w414:dbl, "Lockin 1 Demod 3.Theta (deg)"=w413:dbl)
        n188 = Build Array (concatenate)(w421, w420, w419, w418, w417, w416, w415, w414, w413) -> (w412:dbl[])
      }
    }
    n189 = case shown="True" w361 {
      tunnel: w356 -> [_ w410]
      tunnel: w360 -> [w403 w405]
      tunnel: [w403 w404] -> w358
      frame False {
      }
      frame True {
        n190 = Unbundle By Name(w410) -> ("Lockin 2 Demod 0.R(V)"=w409:dbl, "Lockin 2 Demod 0.Theta (deg)"=w408:dbl, "Lockin 2 Demod 1.R(V)"=w407:dbl, "Lockin 2 Demod 1.Theta (deg)"=w406:dbl)
        n191 = Build Array (concatenate)(w405, w409, w408, w407, w406) -> (w404:dbl[])
      }
    }
    n192 = case shown="False" w359 {
      tunnel: w356 -> [_ w402]
      tunnel: w358 -> [w395 w397]
      tunnel: [w395 w396] -> w355
      frame False {
      }
      frame True {
        n193 = Unbundle By Name(w402) -> ("Lockin 3 Demod 0.R(V)"=w401:dbl, "Lockin 3 Demod 0.Theta (deg)"=w400:dbl, "Lockin 3 Demod 1.R(V)"=w399:dbl, "Lockin 3 Demod 1.Theta (deg)"=w398:dbl)
        n194 = Build Array (concatenate)(w397, w401, w400, w399, w398) -> (w396:dbl[])
      }
    }
    n195 = global read "MQM Data Transfer_KM.vi" "ZI HFLI"() -> (w344:T12)
    n196 = case shown="False" w357 {
      tunnel: w356 -> [_ w394]
      tunnel: w355 -> [w387 w389]
      tunnel: [w387 w388] -> w342
      frame False {
      }
      frame True {
        n197 = Unbundle By Name(w394) -> ("Lockin 4 Demod 0.R(V)"=w393:dbl, "Lockin 4 Demod 0.Theta (deg)"=w392:dbl, "Lockin 4 Demod 1.R(V)"=w391:dbl, "Lockin 4 Demod 1.Theta (deg)"=w390:dbl)
        n198 = Build Array (concatenate)(w389, w393, w392, w391, w390) -> (w388:dbl[])
      }
    }
    n199 = Unbundle By Name(w344) -> ("LI1 active"=w345:bool)
    n200 = case shown="True" w345 {
      tunnel: w344 -> [_ w382]
      tunnel: w342 -> [w374 w375]
      tunnel: [w374 w377] -> w343
      frame False {
      }
      frame True {
        n201 = Unbundle By Name(w382) -> ("Lockin 1 Demod 0.Frequency (Hz)"=w381:dbl, "Lockin 1 Demod 0.R(V)"=w380:dbl, "Lockin 1 Demod 0.Theta (deg)"=w379:dbl, "Lockin 1 Demod 0.X (mV)"=w378:dbl, "Lockin 1 Demod 0.Y (mV)"=w376:dbl)
        n202 = Build Array (concatenate)(w375, w381, w380, w379, w378, w376) -> (w377:dbl[])
      }
    }
    n203 = global read "MQM Data Transfer_KM.vi" "Keithley"() -> (w349:cluster{"Value":dbl, "Keithley on":bool})
    n204 = Unbundle By Name(w349) -> ("Value"=w348:dbl, "Keithley on"=w346:bool)
    n205 = case shown="False" w346 {
      tunnel: w343 -> [w383 w386]
      tunnel: w348 -> [_ w385]
      tunnel: [w383 w384] -> w347
      frame False {
      }
      frame True {
        n206 = Build Array (concatenate)(w386, w385) -> (w384:dbl[])
      }
    }
    n207 = Build Array (concatenate)(w351, w347) -> (w350:dbl[][])
    n208 = flat-sequence {
      tunnel: "Display Elements" -> [w425]
      tunnel: [w429] -> w369
      tunnel: w365 -> [w423]
      tunnel: w350 -> [w424]
      tunnel: w369 -> [w482]
      frame #0 {
        n209 = for {
          tunnel: w425 -> [w462] mode=indexing
          shift-right: [w468] -> w435
          shift-left: dbl[] [] -> [w467]
          shift-right: [w456] -> w433
          shift-left: dbl[][] [] -> [w464]
          shift-right: [w460] -> w429
          shift-left: string[] [] -> [w459]
          tunnel: w423 -> [w455]
          tunnel: w424 -> [w457]
          i -> [w458]
          n210 = Unbundle By Name(w462) -> ("X"=w463:bool, "Y"=w466:bool, "Name"=w461:u16)
          n211 = Index Array(array=w457, index (col)=w461) -> (element=w465:dbl[])  [unwired: 1 in]
          n212 = Select(t=w465, s=w463, f=w467) -> (s? t:f=w468:dbl[])
          n213 = case shown="True" w463 {
            tunnel: w461 -> [_ w471]
            tunnel: w458 -> [_ _]
            tunnel: w455 -> [_ w469]
            frame False {
            }
            frame True {
              n214 = Index Array(array=w469, index=w471) -> (element=w470:string)
              n215 = property on="XY Graph" class="XYGraph (strict)"("XScale.NameLbl.Text"=w470) -> ()  [unwired: 2 in, 2 out]
            }
          }
          n216 = case shown="True" w466 {
            tunnel: w465 -> [_ w474]
            tunnel: w464 -> [w472 w481]
            tunnel: [w472 w480] -> w456
            tunnel: w461 -> [_ w479]
            tunnel: [w473 w477] -> w460
            tunnel: w459 -> [w473 w476]
            tunnel: w455 -> [_ w475]
            frame False {
            }
            frame True {
              n217 = Build Array (concatenate)(w481, w474) -> (w480:dbl[][])
              n218 = Index Array(array=w475, index=w479) -> (element=w478:string)
              n219 = Build Array (concatenate)(w476, w478) -> (w477:string[])
            }
          }
        }
        n220 = Array Size(array=w433) -> (size(s)=w432:i32[])
        n221 = for {
          tunnel: w433 -> [w439] mode=indexing
          tunnel: w435 -> [w441]
          tunnel: [w442] -> w434 mode=indexing
          n222 = case shown="2" "X-Axis" {
            tunnel: w441 -> [w449 w451 w454]
            tunnel: [w449 w450 w453] -> w440
            frame 0, Default {
            }
            frame 1 {
              n223 = Reciprocal(x=w451) -> (1/x=w450:dbl[])
            }
            frame 2 {
              n224 = Absolute Value(x=w454) -> (abs(x)=w452:dbl[])
              n225 = Logarithm Base 10(1:w452) -> (0:w453:dbl[])
            }
          }
          n226 = case shown="0, Default" "Y-Axis" {
            tunnel: w439 -> [w443 w445 w448]
            tunnel: [w443 w444 w447] -> w436
            frame 0, Default {
            }
            frame 1 {
              n227 = Reciprocal(x=w445) -> (1/x=w444:dbl[])
            }
            frame 2 {
              n228 = Absolute Value(x=w448) -> (abs(x)=w446:dbl[])
              n229 = Logarithm Base 10(1:w446) -> (0:w447:dbl[])
            }
          }
          n230 = Bundle(w440, w436) -> (w442:cluster{dbl[], dbl[]})  [unwired: 1 in]
        }
        "XY Graph" <- w434
        n231 = Index Array(array=w432, index=0) -> (element=w430:i32)
        n232 = property on="XY Graph" class="XYGraph (strict)"("LegNumRows"=w430) -> ()  [unwired: 2 in, 2 out]
      }
      frame #1 {
        n233 = for {
          tunnel: w482 -> [w483] mode=indexing
          i -> [w484]
          n234 = property on="XY Graph" class="XYGraph (strict)"("Active Plot"=w484, "Plot.Plot Name"=w483) -> ()  [unwired: 2 in, 2 out]
        }
      }
    }
    "Global Stop" <- "Finish"
  }
  n235 = Strip Path(path="Fequency sweep datafile") -> (stripped path=w16:path, name=w20:string)
  n236 = Concatenate Strings(w20, "_1.dat") -> (w17:string)
  n237 = call "ControlHFLI.vi"("Sweep"="Control", "Bandwidth (Hz)"="Bandwidth (Hz)", "Number of Points"="# pts in scan", "Stop (Hz)"="Stop (Hz)", "Start (Hz)"="Start (Hz)") -> ()  [unwired: 7 in]
  n238 = control-ref of="Plot: fragment - filter"() -> (w4:refnum<vi>)
  n239 = control-ref of="Plot: dz/domega"() -> (w3:refnum<vi>)
  n240 = control-ref of="Plot: fragment"() -> (w8:refnum<vi>)
  n241 = control-ref of="Plot: win omega"() -> (w6:refnum<vi>)
  n242 = control-ref of="Plot: phase around center"() -> (w7:refnum<vi>)
  n243 = control-ref of="Plot: phase"() -> (w5:refnum<vi>)
  n244 = control-ref of="Plot: complex plane"() -> (w9:refnum<vi>)
  n245 = control-ref of="Plot: complex plane - filter"() -> (w10:refnum<vi>)
  n246 = Bundle By Name(cluster=T7 {"Plot: complex plane - filter"=refnum, "Plot: dz/domega"=refnum, "Plot: fragment filter"=refnum, "Plot: win omega"=refnum, "Plot: phase"=refnum, "Plot: phase around center"=refnum, "Plot: complex plane"=refnum, "Plot: fragment"=refnum} ("plots: filter related"), "Plot: complex plane - filter"=w10, "Plot: dz/domega"=w3, "Plot: fragment filter"=w4, "Plot: win omega"=w6, "Plot: phase"=w5, "Plot: phase around center"=w7, "Plot: complex plane"=w9, "Plot: fragment"=w8) -> (w2:T7)
  n247 = while {
    shift-right: [w498] -> _
    shift-left: w17 -> [w508]
    tunnel: w16 -> [w497]
    tunnel: w2 -> [w487]
    stop <- "Stop" continue-if-true
    (unwired) FALSE ("Save current freq scan")
    w510 = dbl[] []
    w513 = dbl[] []
    n248 = Tick Count (ms)() -> (millisecond timer value=w512:u32)
    n249 = while {
      shift-right: [w534] -> w496
      shift-left: w513 -> [w532]
      shift-right: [w535] -> w495
      shift-left: w513 -> [w531]
      shift-right: [w556] -> _
      shift-left: _ -> [w557]
      tunnel: [w559] -> _
      tunnel: w512 -> [w551]
      shift-right: [w530] -> _
      shift-left: 0 -> [w549]
      shift-right: [w539] -> w494
      shift-left: w510 -> [w538]
      shift-right: [w537] -> w493
      shift-left: w510 -> [w540]
      i -> [w536]
      stop <- w533 continue-if-true
      n250 = global read "MQM Data Transfer_KM.vi" "ZI HFLI"() -> (w562:T12)
      n251 = Wait (ms)(milliseconds to wait="DAQ time (ms)") -> ()  [unwired: 1 out]
      n252 = Tick Count (ms)() -> (millisecond timer value=w553:u32)
      n253 = Unbundle By Name(w562) -> ("Lockin 1 Demod 0.Frequency (Hz)"=w556:dbl, "Lockin 1 Demod 0.Theta (deg)"=w558:dbl)
      n254 = Subtract(x=w553, y=w551) -> (x-y=w530:u32)
      n255 = global read "MQM Data Transfer_KM.vi" "ZI HFLI"() -> (w544:T12)
      n256 = Subtract(x=w530, y=w549) -> (x-y=→"Data Rate  (ms)":u32)
      n257 = Unbundle By Name(w544) -> ("Lockin 1 Demod 0.X (mV)"=w542:dbl, "Lockin 1 Demod 0.Y (mV)"=w541:dbl)
      n258 = Add(x=w556, y=1) -> (x+y=w555:dbl)
      n259 = Build Array (concatenate)(w531, w556) -> (w564:dbl[])
      n260 = Greater?(x=w555, y=w557) -> (0:w533:bool)
      n261 = Build Array (concatenate)(w532, w558) -> (w563:dbl[])
      n262 = case shown="2" "Frequency" {
        tunnel: w564 -> [w585 w587 w590]
        tunnel: [w585 w586 w589] -> w535
        frame 0, Default {
        }
        frame 1 {
          n263 = Reciprocal(x=w587) -> (1/x=w586:dbl[])
        }
        frame 2 {
          n264 = Absolute Value(x=w590) -> (abs(x)=w588:dbl[])
          n265 = Logarithm Base 10(1:w588) -> (0:w589:dbl[])
        }
      }
      n266 = case shown="0, Default" "Theta" {
        tunnel: [w579 w581 w584] -> w534
        tunnel: w563 -> [w579 w580 w582]
        frame 0, Default {
        }
        frame 1 {
          n267 = Reciprocal(x=w580) -> (1/x=w581:dbl[])
        }
        frame 2 {
          n268 = Absolute Value(x=w582) -> (abs(x)=w583:dbl[])
          n269 = Logarithm Base 10(1:w583) -> (0:w584:dbl[])
        }
      }
      n270 = Build Array (concatenate)(w538, w542) -> (w546:dbl[])
      n271 = Build Array (concatenate)(w540, w541) -> (w545:dbl[])
      n272 = case shown="2" "X" {
        tunnel: w546 -> [w573 w575 w578]
        tunnel: [w573 w574 w577] -> w539
        frame 0, Default {
        }
        frame 1 {
          n273 = Reciprocal(x=w575) -> (1/x=w574:dbl[])
        }
        frame 2 {
          n274 = Absolute Value(x=w578) -> (abs(x)=w576:dbl[])
          n275 = Logarithm Base 10(1:w576) -> (0:w577:dbl[])
        }
      }
      n276 = case shown="0, Default" "Y" {
        tunnel: [w567 w569 w572] -> w537
        tunnel: w545 -> [w567 w568 w570]
        frame 0, Default {
        }
        frame 1 {
          n277 = Reciprocal(x=w568) -> (1/x=w569:dbl[])
        }
        frame 2 {
          n278 = Absolute Value(x=w570) -> (abs(x)=w571:dbl[])
          n279 = Logarithm Base 10(1:w571) -> (0:w572:dbl[])
        }
      }
      n280 = Divide(x=w535, y=1000) -> (x/y=w560:dbl[])
      n281 = Bundle(w560, w534) -> (w559:cluster{dbl[], dbl[]})  [unwired: 1 in]
      "Phase" <- w559
      n282 = Bundle(w539, w537) -> (→"Circles":cluster{dbl[], dbl[]})  [unwired: 1 in]
      "# pts in freq sweep" <- w536
    }
    n283 = local write "Save current freq scan"(FALSE) -> ()
    n284 = case shown="True" "Save current freq scan" {
      tunnel: [w515 w517] -> w498
      tunnel: w508 -> [w515 w516]
      frame False {
      }
      frame True {
        n285 = Search/Split String(string=w516, search string/char (-)="_") -> (substring before match=w528:string, match + rest of string=w527:string)  [unwired: 1 in, 1 out]
        n286 = Decimal String To Number(string=w527, offset=1) -> (number=w525:i32)  [unwired: 1 in, 1 out]
        n287 = Add(x=w525, y=1) -> (x+y=w522:i32)
        n288 = Number To Fractional String(use system decimal point (T)=FALSE, number=w522, precision (6)=0) -> (F-format string=w521:string)  [unwired: 1 in]
        n289 = Concatenate Strings(w528, "_", w521, ".dat") -> (w517:string)
      }
    }
    n290 = call "KM_peak -- find -- pm - V1.vi"("omega in"=w495, "z in"=w494, 2:w493, "parameters: complex fit"="parameters: complex fit", "plots: filter related"=w487, "plot staff ?"="plot staff", "just guess?"="use fast fit?", "subtract linear BG"="subtract linear BG") -> ("good lorentzian"=→"good lorentzian":T1, "pm lorentzian"=→"pm lorentzian":T1, "cp lorentzian"=→"cp lorentzian":T1)  [unwired: 9 in]
    n291 = Build Path(base path=w497, name or relative path=w498) -> (appended path=w506:path)
    n292 = Build Array(w495, w496) -> (w504:dbl[][])
    n293 = Transpose 2D Array(2D array=w504) -> (transposed array=w505:dbl[][])
    n294 = call-poly <vilib>:"Write To Spreadsheet File.vi"("append to file? (new file:F)"=FALSE, "1D data"=string[] ["Frequency (Hz) ", "Theta (deg)"], "file path (dialog if empty)"=w506) -> ("new file path (Not A Path if cancelled)"=w500:path)  [unwired: 5 in]
    n295 = call-poly <vilib>:"Write To Spreadsheet File.vi"("format (%.3f)"="%.8f", "append to file? (new file:F)"=TRUE, "2D data"=w505, "file path (dialog if empty)"=w500) -> ()  [unwired: 4 in, 1 out]
  }
